vi "Measurement_GetMetadata_ContainsExpectedMeasurementDetails.vi"(8 "error in":errorcluster, 10 "expected measurement details":T1, 11 "run service vi":refnum<vi>) -> (0 "error out":errorcluster, 2 "result":string, 3 "pass":bool)   [LabVIEW 2021, in "MeasurementServerTests.lvlib" / "Measurement Service Tests.lvlib"]
uses:
  Measurement Service Tests.lvlib
  gRPC/Generated APIs/ni/measurementlink/measurement/v2/Measurement Service Client V2/RPC Messages/ni_measurementlink_measurement_v2_MeasurementDetails.ctl
  Runtime/Measurements/Helpers/TypeDefs/Measurement Server User Settings.ctl
  Runtime/Measurements/Helpers/TypeDefs/Stop Server User Event.ctl
  Runtime/Measurements/Helpers/TypeDefs/Measurement Service Version.ctl
  97159654-2b8c-44d4-92ef-9b7ec1865e5c.vi
  Runtime/Measurements/NI Measurement Plug-In SDK.lvlib
  Continuous Counting Client/Continuous Counting Client.lvlib
  gRPC/Generated APIs/ni/measurementlink/measurement/v2/Measurement Service Client V2/Measurement Service Client V2.lvlib
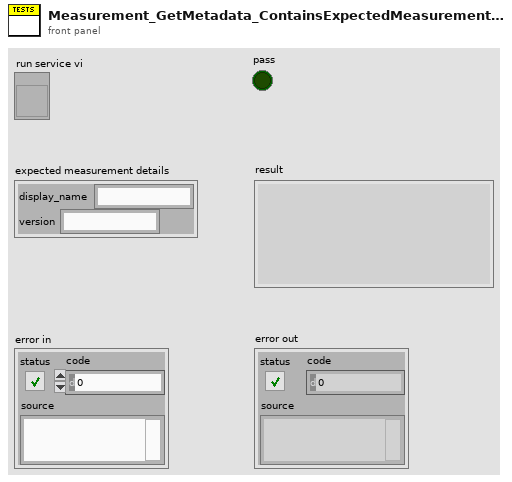
[diagram p1: front panel]
types:
  T1 = typedef "Measurement Service Client V2.lvlib/ni_measurementlink_measurement_v2_MeasurementDetails.ctl" = cluster{"display_name":string, "version":string}
  T2 = typedef "NI Measurement Plug-In SDK.lvlib/Measurement Service Version.ctl" = enum16{"V1", "V2"}
  T3 = typedef "NI Measurement Plug-In SDK.lvlib/Measurement Server User Settings.ctl" = cluster{"stop server":T4, "measurement service versions":T2[]}
  T4 = typedef "NI Measurement Plug-In SDK.lvlib/Stop Server User Event.ctl" = refnum<user-event>
  T5 = typedef "grpc-lvsupport-release.lvlib/grpcId.ctl" = u64
  T6 = typedef "Measurement Service Client V2.lvlib/ni_measurementlink_measurement_v2_GetMetadataResponse.ctl" = cluster{"measurement_details":T1, "measurement_signature":T7, "user_interface_details":T14[]}
  T7 = typedef "Measurement Service Client V2.lvlib/ni_measurementlink_measurement_v2_MeasurementSignature.ctl" = cluster{"configuration_parameters_message_type":string, "configuration_parameters":T8[], "configuration_defaults":T11, "outputs_message_type":string, "outputs":T12[]}
  T8 = typedef "Measurement Service Client V2.lvlib/ni_measurementlink_measurement_v2_ConfigurationParameter.ctl" = cluster{"field_number":i32, "type":T9, "name":string, "repeated":bool, "annotations":T10[], "message_type":string}
  T9 = typedef "Measurement Service Client V2.lvlib/google_protobuf_Field_Kind.ctl" = enum32{"TYPE_UNKNOWN", "TYPE_DOUBLE", "TYPE_FLOAT", "TYPE_INT64", "TYPE_UINT64", "TYPE_INT32", "TYPE_FIXED64", "TYPE_FIXED32", "TYPE_BOOL", "TYPE_STRING", "TYPE_GROUP", "TYPE_MESSAGE", "TYPE_BYTES", "TYPE_UINT32", "TYPE_ENUM", "TYPE_SFIXED32", "TYPE_SFIXED64", "TYPE_SINT32", "TYPE_SINT64"}
  T10 = typedef "Measurement Service Client V2.lvlib/ni_measurementlink_measurement_v2_ConfigurationParameter_AnnotationsEntry.ctl" = cluster{"key":string, "value":string}
  T11 = typedef "Measurement Service Client V2.lvlib/google_protobuf_Any.ctl" = cluster{"type_url":string, "value":u8[]}
  T12 = typedef "Measurement Service Client V2.lvlib/ni_measurementlink_measurement_v2_Output.ctl" = cluster{"field_number":i32, "type":T9, "name":string, "repeated":bool, "annotations":T13[], "message_type":string}
  T13 = typedef "Measurement Service Client V2.lvlib/ni_measurementlink_measurement_v2_Output_AnnotationsEntry.ctl" = cluster{"key":string, "value":string}
  T14 = typedef "Measurement Service Client V2.lvlib/ni_measurementlink_measurement_v2_UserInterfaceDetails.ctl" = cluster{"file_url":string}
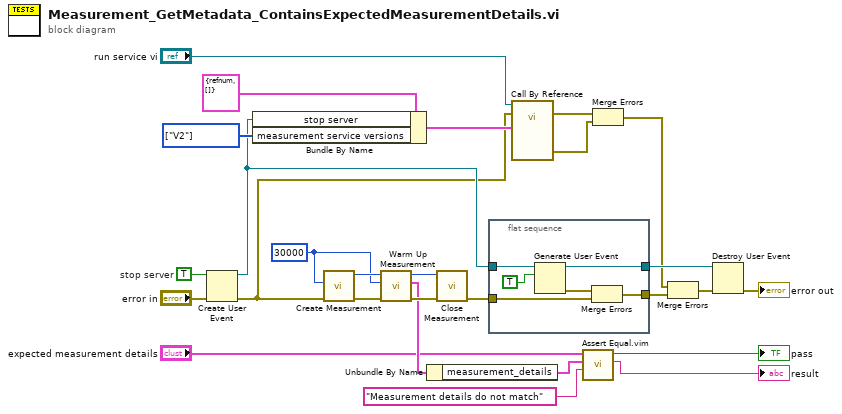
[diagram p0: block diagram]
diagram:
  w19 = 30000 ("ms timeout")
  w25 = TRUE  # stop server
  w26 = T2[] [enum."V2"] items=["V1", "V2"] ("measurement service versions")
  n1 = Create User Event(user event datatype=w25, error in="error in") -> (user event=w23:refnum<user-event>, error out=w12:errorcluster)
  n2 = Bundle By Name(cluster=T3 {"stop server"=refnum, "measurement service versions"=[]} ("server settings"), "stop server"=w23, "measurement service versions"=w26) -> (w13:T3)
  n3 = call "Create Measurement.vi"("error in"=w12, "ms timeout"=w19) -> ("error out"=w21:errorcluster, "gRPCid out"=w20:T5)  [unwired: 8 in]
  n4 = call "Warm Up Measurement.vi"("error in"=w21, "timeout (ms)"=w19, "gRPC ID"=w20) -> ("error out"=w7:errorcluster, "get metadata response"=w6:T6, "gRPC ID out"=w8:T5)  [unwired: 6 in]
  n5 = Unbundle By Name(w6) -> ("measurement_details"=w5:T1)
  n6 = call "Close Measurement.vi"("error in"=w7, "gRPCid in"=w8) -> ("error out"=w22:errorcluster)  [unwired: 9 in]
  n7 = flat-sequence {
    tunnel: w23 -> [w32]
    tunnel: [w31] -> w16
    tunnel: [w30] -> w18
    tunnel: w22 -> [w29]
    frame #0 {
      n8 = Generate User Event(user event=w32, event data cluster=TRUE ("event data")) -> (user event out=w31:refnum<user-event>, error out=w33:errorcluster)  [unwired: 2 in]
      n9 = Merge Errors(w33, w29) -> (w30:errorcluster)
    }
  }
  n10 = call-by-ref "?"(reference="run service vi", error in=w12, "server settings"=w13) -> (error out=w14:errorcluster, 0:"error out"=w9:errorcluster)  [unwired: 10 in, 1 out]
  n11 = call "Assert Equal.vim"("failure message"="Measurement details do not match", "actual value"=w5, "expected value"="expected measurement details") -> ("message"=→"result":string, "equal?"=→"pass":bool)  [unwired: 7 in]
  n12 = Merge Errors(w14, w9) -> (w10:errorcluster)
  n13 = Merge Errors(w10, w18) -> (w17:errorcluster)
  n14 = Destroy User Event(user event=w16, error in=w17) -> (error out=→"error out":errorcluster)
